vi "Some VI.vi"(8 "Error In":errorcluster) -> (0 "Error Out":errorcluster, 2 "signal out 2":waveform(dbl), 3 "Numeric":fxp<+,16,16>, 5 "String":string)   [LabVIEW 2014]
uses:
  <vilib>/measure/NI_MABase.lvlib
panel:
  out "signal out 3":waveform(dbl)
  out "signal out":waveform(dbl)
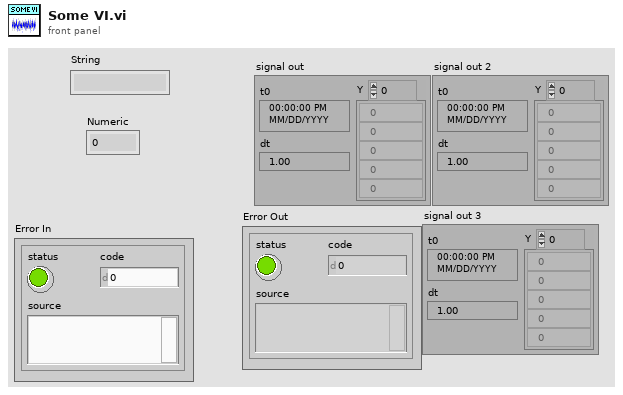
[diagram p1: front panel]
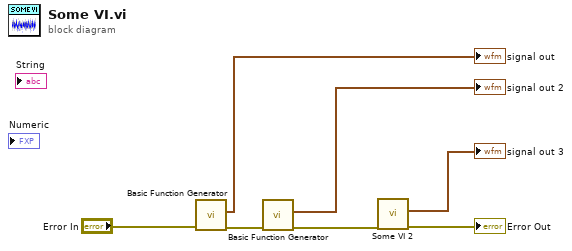
[diagram p0: block diagram]
diagram:
  n1 = call <vilib>:"Basic Function Generator.vi"("error in (no error)"="Error In") -> ("error out"=w6:errorcluster, "signal out"=→"signal out":waveform(dbl))  [unwired: 8 in, 1 out]
  n2 = call <vilib>:"Basic Function Generator.vi"("error in (no error)"=w6) -> ("error out"=w3:errorcluster, "signal out"=→"signal out 2":waveform(dbl))  [unwired: 8 in, 1 out]
  n3 = call "Some VI 2.vi"("Error In"=w3) -> ("Error Out"=→"Error Out":errorcluster, "signal out 2"=→"signal out 3":waveform(dbl))  [unwired: 9 in]
